vi "Config.vi"(8 "error in (no error)":errorcluster, 10 "Setting":T1={"Max. Volt"=10.0, "Current Limit"=0.5, "Volt Level"=10.0}, 11 "APS7050 in":refnum<class "APS7050.lvclass">) -> (0 "error out":errorcluster, 3 "APS7050 out":refnum<class "APS7050.lvclass">)   [LabVIEW 2019, in "Concrete.lvlib" / "APS7050.lvclass"]
uses:
  APS7050.lvclass
  APS7050.lvclass/APS7050.ctl
  <instrlib>/APS-7000 Series/APS-7000 Series.lvlib
panel:
  in  "Additional Setting":T2
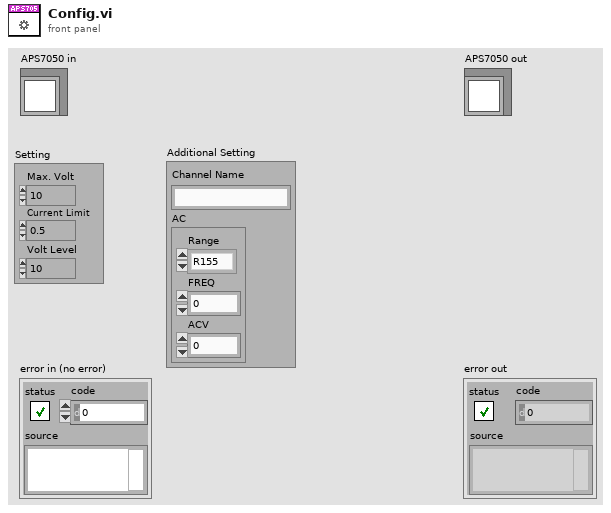
[diagram p1: front panel]
types:
  T1 = cluster{"Max. Volt":dbl, "Current Limit":dbl, "Volt Level":dbl}
  T2 = cluster{"Channel Name":string, "AC":cluster{"Range":enum16{"R155", "R310", "R600", "AUTO"}, "FREQ":dbl, "ACV":dbl}}
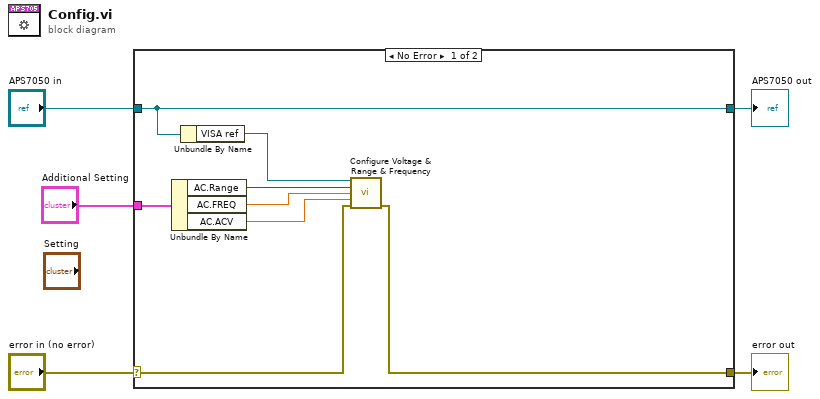
[diagram p0: block diagram]
diagram:
  n1 = case shown="No Error" "error in (no error)" {
    selector: "error in (no error)" -> [w12 w15]
    tunnel: [w11 w15] -> w4
    tunnel: [w7 w14] -> w2
    tunnel: "APS7050 in" -> [w7 w14]
    tunnel: "Additional Setting" -> [w13 _]
    frame No Error {
      n2 = Unbundle By Name(w13) -> ("AC.Range"=w10:enum16{"R155", "R310", "R600", "AUTO"}, "AC.FREQ"=w9:dbl, "AC.ACV"=w8:dbl)
      n3 = Unbundle By Name(w7) -> ("VISA ref"=w6:refnum<visa-resource-name>)
      n4 = call <instrlib>:"Configure Voltage & Range & Frequency.vi"("VISA in"=w6, "Range"=w10, "FREQ"=w9, "ACV"=w8, "error in"=w12) -> ("error out"=w11:errorcluster)  [unwired: 2 in, 8 out]
    }
    frame Error {
    }
  }
  "error out" <- w4
  "APS7050 out" <- w2
